vi "oax_gsGetting Started with OAT Introduction.vi"() -> ()   [LabVIEW 2017]
panel:
  in  "String":string="         Getting Started with Order Analysis Demo Introduction\n\nThe NI Sound and Vibration Measurement Suite provides Order Analysis VIs for analyzing sound or vibration signals generated by rotating or reciprocating machinery, such as engines, compressors, turbines, and pumps. With the Order Analysis VIs, you can reduce sound or vibration signals to meaningful formats, separate rotational and structural components, associate signal components with specific mechanical parts, and perform repeatable measurements. You mainly use Order Analysis VIs in noise, vibration and harshness (NVH) testing as well as machine condition monitoring (MCM) applications.\n\nGetting Started with Order Analysis Demo VI shows most of the order analysis functions. This loads pre-stored data and simulates the online processing repeatedly. The order analysis functions this VI displays are: Speed Profile, Colormap, Waterfall Graph, Cascade Plot, Order Power Spectrum, Order Magnitude and Phase, Polar Plot, Orbit Plot, Timebase Plot, and Shaft Centerline Plot. The Orbit Plot, Timebase Plot and Shaft Centerline Plot are specifically for MCM applications. The other functions are for both NVH and MCM applications. All the functions in this VI use resampling-based order analysis method. You can use these functions to perform order analysis in both online and offline applications.\n"
  in  "STOP":bool
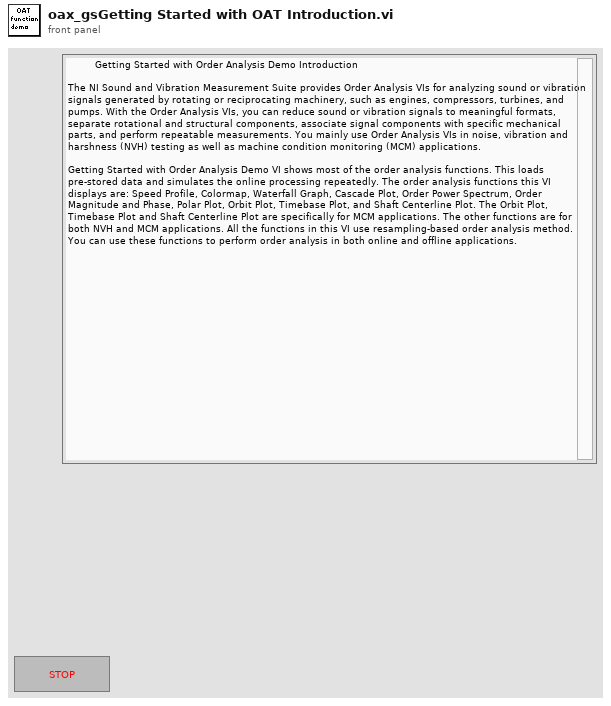
[diagram p1: front panel]
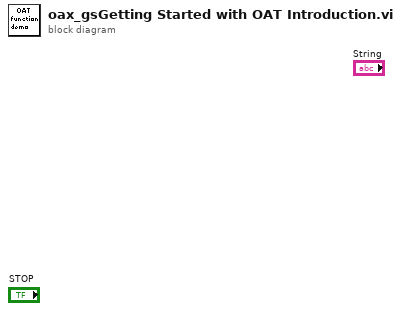
[diagram p0: block diagram]
diagram:
